vi "CRYCal Harmonics IM.vi"(0 "HT Option":bool[](array[boolean]), 1 "x":dbl[](array[numeric]), 2 "z":dbl[](array[numeric]), 3 "Index":i32, 5 "Method":u16, 7 "Harmonic":dbl[](array[numeric]), 9 "Freq resp curves":dbl[][](array[numeric]), 11 "Total Noise":dbl[](array[numeric]), 12 "Fs":dbl format="%.2f", 13 "max value1":dbl, 14 "max value2":dbl) -> (4 "Harmonic Track Out":T1(array[cluster]))   [LabVIEW 2013]
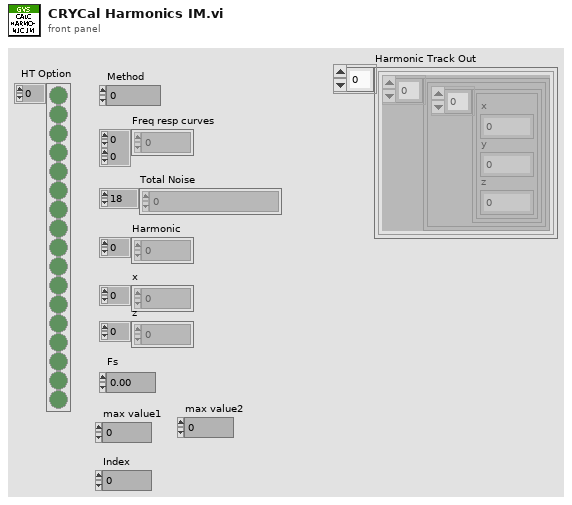
[diagram p1: front panel]
types:
  T1 = cluster{cluster{cluster{"x":dbl, "y":dbl, "z":dbl}[]}[]}[]
  T2 = cluster{"Freq resp curves clipped":cluster{cluster{"x":dbl, "y":dbl, "z":dbl}[]}[]}[]
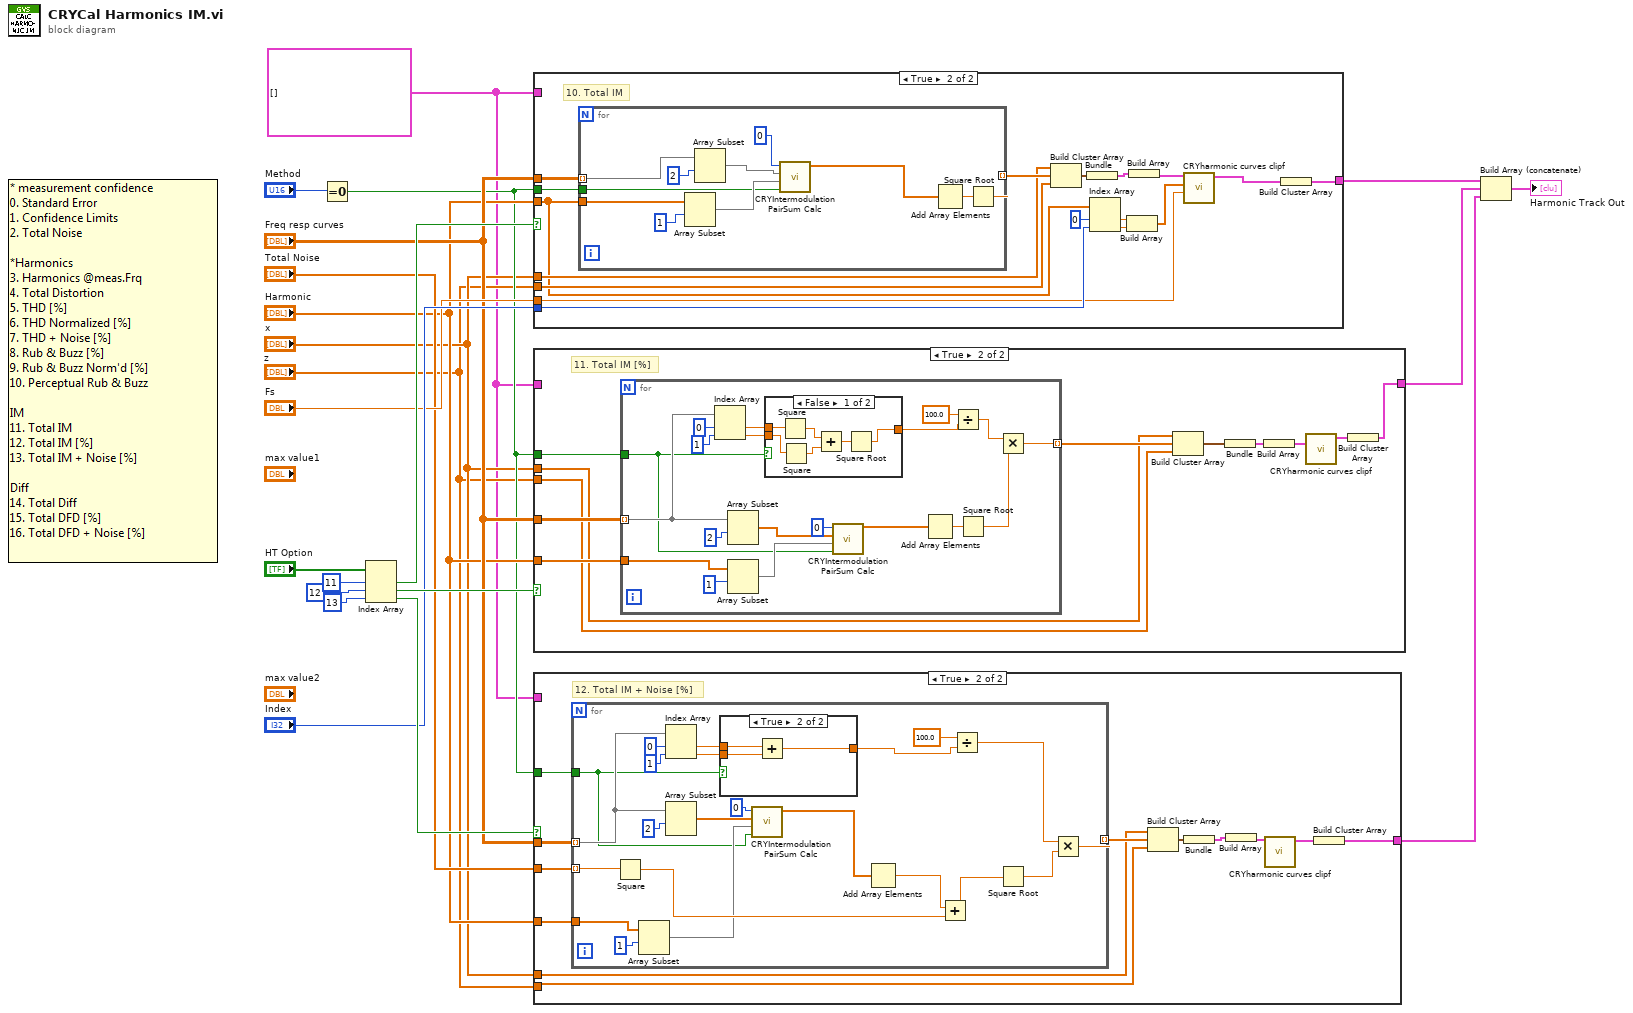
[diagram p0: block diagram]
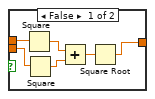
[diagram p3: hidden frame]
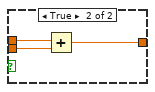
[diagram p5: hidden frame]
diagram:
  w4 = cluster{cluster{cluster[]}[]}[] []
  n1 = Equal To 0?(x="Method") -> (x = 0?=w7:bool)
  n2 = Index Array(array="HT Option", index #1=11 ("index"), index #2=12 ("index"), index #3=13 ("index")) -> (element #1=w15:bool, element #2=w14:bool, element #3=w13:bool)
  n3 = case shown="True" w15 {
    tunnel: [w22 w34] -> w3
    tunnel: "Freq resp curves" -> [_ w33]
    tunnel: w7 -> [_ w32]
    tunnel: "Harmonic" -> [_ w25]
    tunnel: "x" -> [_ w31]
    tunnel: "z" -> [_ w30]
    tunnel: "Index" -> [_ w26]
    tunnel: "Fs" -> [_ w23]
    tunnel: w4 -> [w22 _]
    frame False {
    }
    frame True {
      # "10. Total IM"
      n4 = for {
        tunnel: w33 -> [w48] mode=indexing
        tunnel: [w45] -> w37 mode=indexing
        tunnel: w25 -> [w40]
        tunnel: w32 -> [w41]
        n5 = Array Subset(array=w40, index=1) -> (w43:dbl[])  [unwired: 1 in]
        n6 = Array Subset(array=w48, index=2) -> (w44:dbl[])  [unwired: 1 in]
        n7 = call "CRYIntermodulation PairSum Calc.vi"("Is IEC?"=w41, "Order Array"=w43, "Data Array"=w44, "Type"=u32 0) -> ("PairSum Array"=w46:dbl[])  [unwired: 7 in]
        n8 = Add Array Elements(numeric array=w46) -> (sum=w50:dbl)
        n9 = Square Root(x=w50) -> (sqrt(x)=w45:dbl)
      }
      n10 = Build Cluster Array(w31, w37, w30) -> (w38:cluster{"x":dbl, dbl, "Z":dbl}[])
      n11 = Bundle(w38) -> (w39:cluster{cluster{"x":dbl, dbl, "Z":dbl}[]})  [unwired: 1 in]
      n12 = Index Array(array=w25, index #1=0 ("Index"), index #2=w26) -> (element #1=w28:dbl, element #2=w27:dbl)
      n13 = Build Array(w28, w27) -> (w24:dbl[])
      n14 = Build Array(w39) -> (w36:cluster{cluster{"x":dbl, dbl, "Z":dbl}[]}[])
      n15 = call "CRYharmonic curves clipf.vi"("Fs"=w23, "Harmonics"=w24, "Freq resp curves"=w36) -> ("Freq resp curves clipped"=w35:cluster{cluster{"x":dbl, "y":dbl, "z":dbl}[]}[])  [unwired: 8 out]
      n16 = Build Cluster Array(w35) -> (w34:T2)
    }
  }
  n17 = case shown="True" w14 {
    tunnel: "Freq resp curves" -> [_ w57]
    tunnel: "Harmonic" -> [_ w56]
    tunnel: w7 -> [_ w55]
    tunnel: w4 -> [w51 _]
    tunnel: [w51 w54] -> w2
    tunnel: "z" -> [_ w52]
    tunnel: "x" -> [_ w53]
    frame False {
    }
    frame True {
      # "11. Total IM [%]"
      n18 = for {
        tunnel: w57 -> [w77] mode=indexing
        tunnel: [w68] -> w61 mode=indexing
        tunnel: w56 -> [w81]
        tunnel: w55 -> [w63]
        n19 = Index Array(array=w77, index #1=0 ("index"), index #2=1 ("index")) -> (element #1=w74:dbl, element #2=w73:dbl)
        n20 = Array Subset(array=w77, index=2) -> (w66:dbl[])  [unwired: 1 in]
        n21 = Array Subset(array=w81, index=1) -> (w65:dbl[])  [unwired: 1 in]
        n22 = case shown="False" w63 {
          tunnel: w74 -> [w87 w90]
          tunnel: w73 -> [w86 w89]
          tunnel: [w82 w88] -> w72
          frame False {
            n23 = Square(x=w87) -> (x^2=w85:dbl)
            n24 = Square(x=w86) -> (x^2=w84:dbl)
            n25 = Add(x=w85, y=w84) -> (x+y=w83:dbl)
            n26 = Square Root(x=w83) -> (sqrt(x)=w82:dbl)
          }
          frame True {
            n27 = Add(x=w90, y=w89) -> (x+y=w88:dbl)
          }
        }
        n28 = call "CRYIntermodulation PairSum Calc.vi"("Is IEC?"=w63, "Order Array"=w65, "Data Array"=w66, "Type"=u32 0) -> ("PairSum Array"=w67:dbl[])  [unwired: 7 in]
        n29 = Add Array Elements(numeric array=w67) -> (sum=w80:dbl)
        n30 = Divide(x=100.0, y=w72) -> (x/y=w69:dbl)
        n31 = Square Root(x=w80) -> (sqrt(x)=w70:dbl)
        n32 = Multiply(x=w69, y=w70) -> (x*y=w68:dbl)
      }
      n33 = Build Cluster Array(w53, w61, w52) -> (w62:cluster{"x":dbl, dbl, "Z":dbl}[])
      n34 = Bundle(w62) -> (w60:cluster{cluster{"x":dbl, dbl, "Z":dbl}[]})  [unwired: 1 in]
      n35 = Build Array(w60) -> (w59:cluster{cluster{"x":dbl, dbl, "Z":dbl}[]}[])
      n36 = call "CRYharmonic curves clipf.vi"("Freq resp curves"=w59) -> ("Freq resp curves clipped"=w58:cluster{cluster{"x":dbl, "y":dbl, "z":dbl}[]}[])  [unwired: 2 in, 8 out]
      n37 = Build Cluster Array(w58) -> (w54:T2)
    }
  }
  n38 = case shown="True" w13 {
    tunnel: [w91 w101] -> w1
    tunnel: "Freq resp curves" -> [_ w97]
    tunnel: "Total Noise" -> [_ w96]
    tunnel: "Harmonic" -> [_ w95]
    tunnel: w7 -> [_ w94]
    tunnel: "x" -> [_ w93]
    tunnel: "z" -> [_ w92]
    tunnel: w4 -> [w91 _]
    frame False {
    }
    frame True {
      # "12. Total IM + Noise [%]"
      n39 = for {
        tunnel: w97 -> [w122] mode=indexing
        tunnel: [w116] -> w100 mode=indexing
        tunnel: w95 -> [w125]
        tunnel: w96 -> [w115] mode=indexing
        tunnel: w94 -> [w104]
        n40 = Square(x=w115) -> (x^2=w113:dbl)
        n41 = Array Subset(array=w125, index=1) -> (w109:dbl[])  [unwired: 1 in]
        n42 = Index Array(array=w122, index #1=0 ("index"), index #2=1 ("index")) -> (element #1=w107:dbl, element #2=w106:dbl)
        n43 = Array Subset(array=w122, index=2) -> (w110:dbl[])  [unwired: 1 in]
        n44 = case shown="True" w104 {
          tunnel: w107 -> [w131 w134]
          tunnel: w106 -> [w130 w133]
          tunnel: [w126 w132] -> w105
          frame False {
            n45 = Square(x=w131) -> (x^2=w129:dbl)
            n46 = Square(x=w130) -> (x^2=w128:dbl)
            n47 = Add(x=w129, y=w128) -> (x+y=w127:dbl)
            n48 = Square Root(x=w127) -> (sqrt(x)=w126:dbl)
          }
          frame True {
            n49 = Add(x=w134, y=w133) -> (x+y=w132:dbl)
          }
        }
        n50 = call "CRYIntermodulation PairSum Calc.vi"("Is IEC?"=w104, "Order Array"=w109, "Data Array"=w110, "Type"=u32 0) -> ("PairSum Array"=w111:dbl[])  [unwired: 7 in]
        n51 = Add Array Elements(numeric array=w111) -> (sum=w114:dbl)
        n52 = Add(x=w114, y=w113) -> (x+y=w112:dbl)
        n53 = Divide(x=100.0, y=w105) -> (x/y=w117:dbl)
        n54 = Square Root(x=w112) -> (sqrt(x)=w118:dbl)
        n55 = Multiply(x=w117, y=w118) -> (x*y=w116:dbl)
      }
      n56 = Build Cluster Array(w93, w100, w92) -> (w102:cluster{"x":dbl, dbl, "Z":dbl}[])
      n57 = Bundle(w102) -> (w103:cluster{cluster{"x":dbl, dbl, "Z":dbl}[]})  [unwired: 1 in]
      n58 = Build Array(w103) -> (w99:cluster{cluster{"x":dbl, dbl, "Z":dbl}[]}[])
      n59 = call "CRYharmonic curves clipf.vi"("Freq resp curves"=w99) -> ("Freq resp curves clipped"=w98:cluster{cluster{"x":dbl, "y":dbl, "z":dbl}[]}[])  [unwired: 2 in, 8 out]
      n60 = Build Cluster Array(w98) -> (w101:T2)
    }
  }
  n61 = Build Array (concatenate)(w3, w2, w1) -> (→"Harmonic Track Out":T2)
